vi "query.vi"(0 "object in":refnum<class "access_work.lvclass">, 1 "database":string(combo), 2 "table输入":string(combo), 3 "columns":string[](array[string]), 4 "condition":string, 5 "error in (no error)":errorcluster) -> (14 "object out":refnum<class "access_work.lvclass">, 15 "data":string[][](table), 16 "columns输出":string[](array[string]), 17 "拆分数据":bool, 19 "error out":errorcluster)   [LabVIEW 2016, in "access_work.lvclass"]
uses:
  access_work.lvclass
  <vilib>/Utility/sysdir.llb/System Directory Type.ctl
  <vilib>/addons/database/Connection.llb/DB Tools Open Connec (String).vi
  <vilib>/addons/database/_DB Variant To Data/Database Variant To Data.xnode
  <vilib>/addons/database/NI_Database_API.lvlib
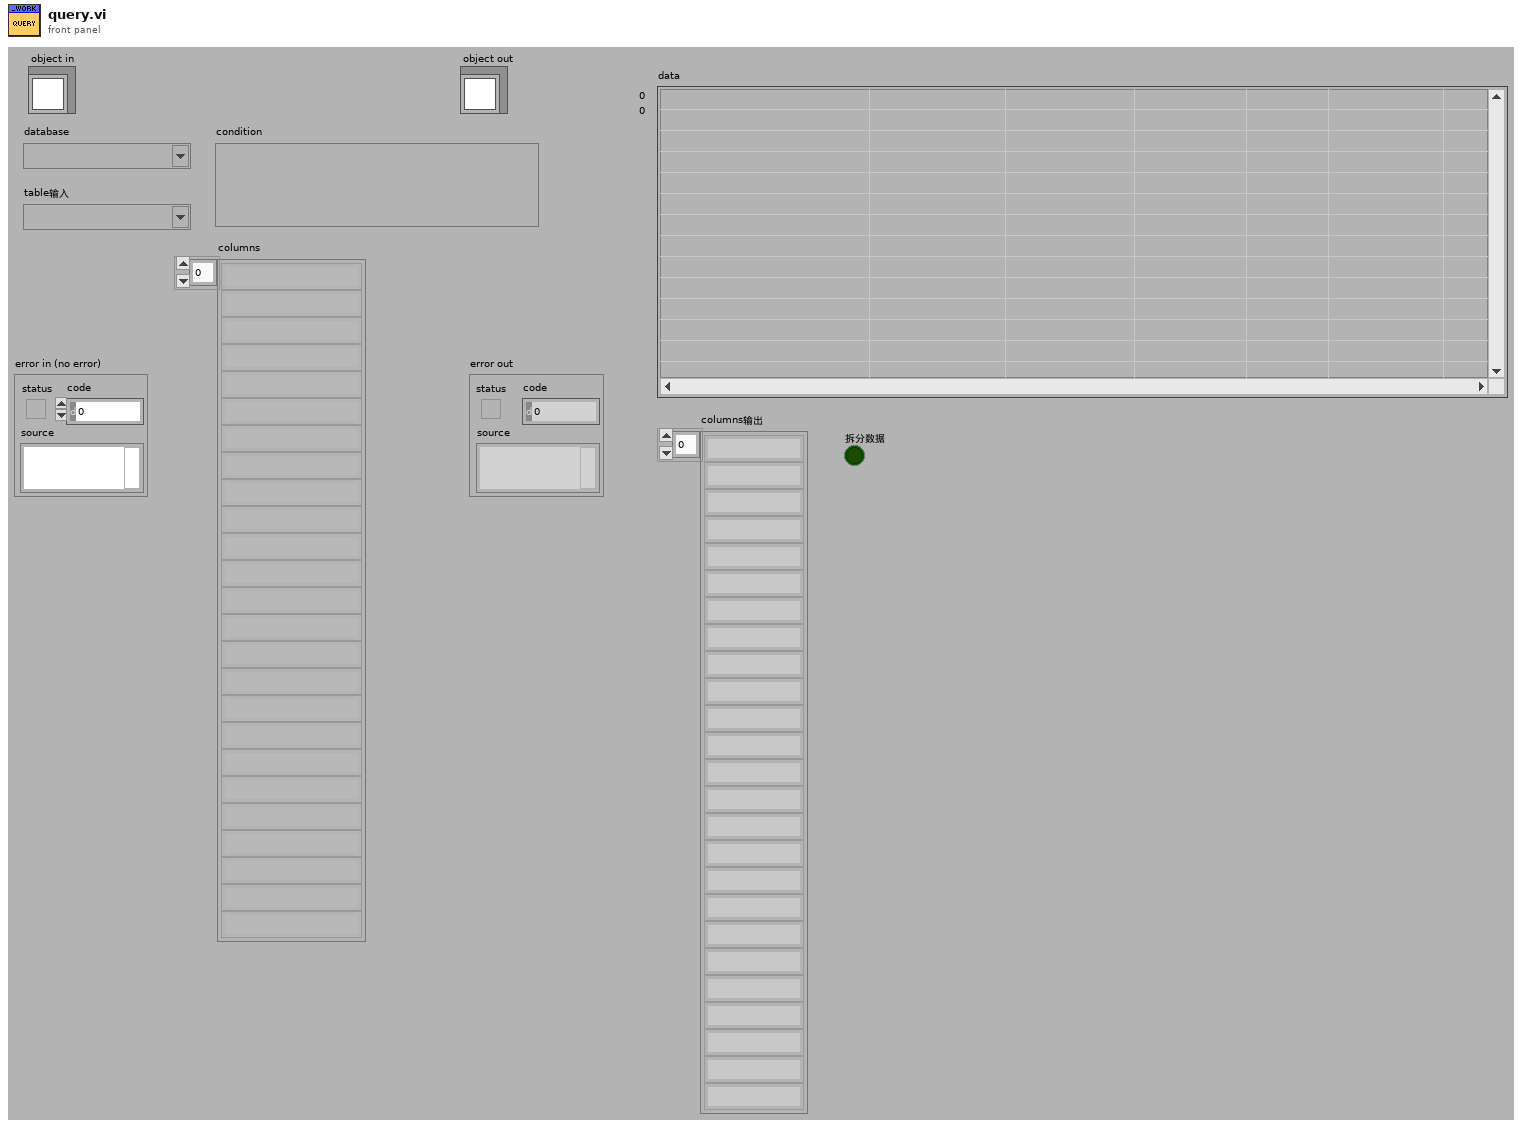
[diagram p1: front panel]
types:
  T1 = typedef "System Directory Type.ctl" = i32
  T2 = typedef "NI_Database_API.lvlib/Conn ObjectReference.ctl" = refnum<k1>
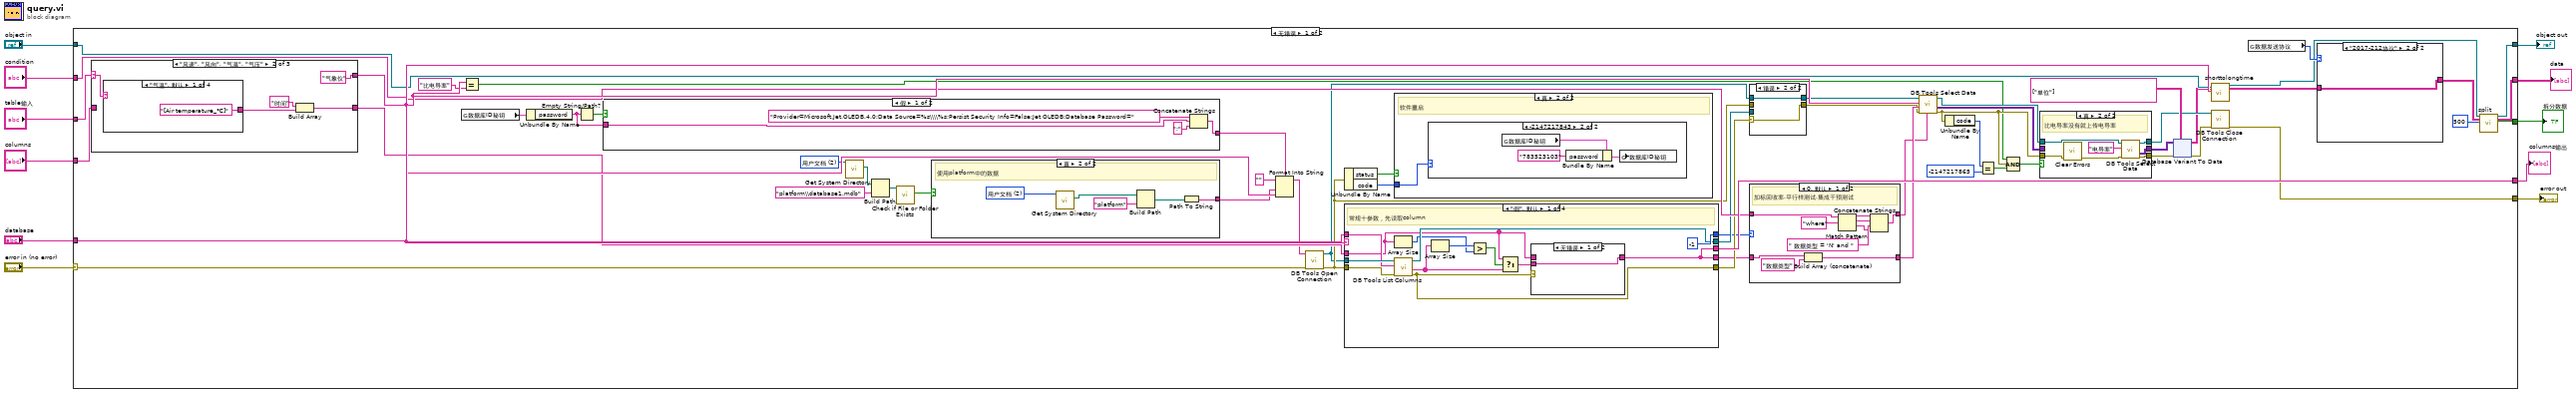
[diagram p0: block diagram]
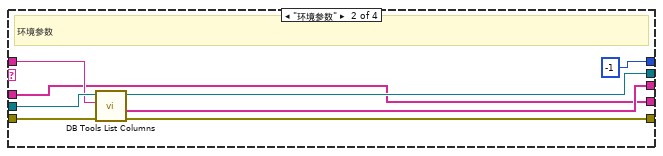
[diagram p6: hidden frame]
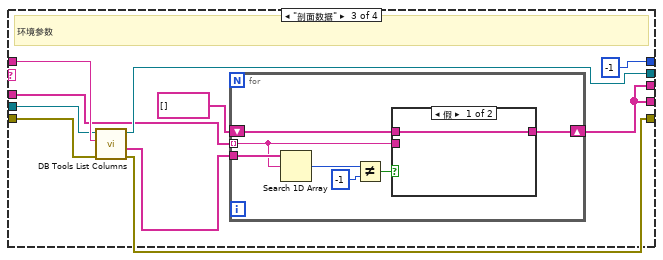
[diagram p7: hidden frame]
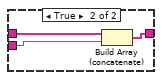
[diagram p8: hidden frame]
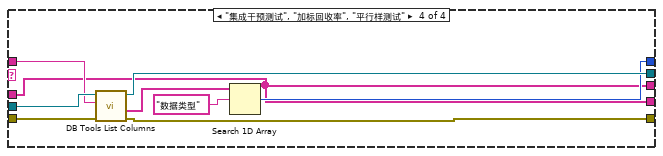
[diagram p9: hidden frame]
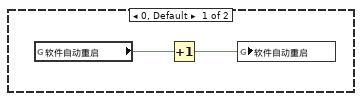
[diagram p11: hidden frame]
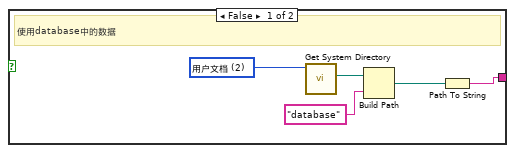
[diagram p12: hidden frame]
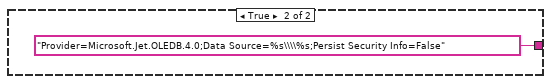
[diagram p13: hidden frame]
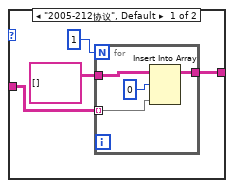
[diagram p14: hidden frame]
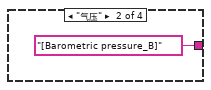
[diagram p16: hidden frame]
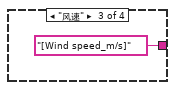
[diagram p17: hidden frame]
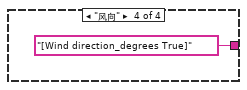
[diagram p18: hidden frame]
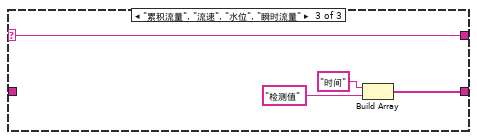
[diagram p19: hidden frame]
diagram:
  n1 = case shown="无错误" "error in (no error)" {
    selector: "error in (no error)" -> [w64 w238]
    tunnel: [w60 w238] -> w10
    tunnel: [w53 w237] -> w8
    tunnel: "object in" -> [w59 w237]
    tunnel: "table输入" -> [w68 _]
    tunnel: "columns" -> [w67 _]
    tunnel: "database" -> [w65 _]
    tunnel: [w63 _] -> w4
    tunnel: "condition" -> [w61 _]
    tunnel: [w52 _] -> w2
    tunnel: [w51 _] -> w1
    frame No Error {
      w45 = T1 2 items=["用户目录"=0, "用户桌面"=1, "用户文档"=2, "用户应用程序数据"=3, "用户设置"=4, "用户临时目录"=5, "公共文档"=6, "公共应用程序数据"=7, "公共设置"=8, "公共缓存"=13, "系统核心库"=9, "系统安装库"=10, "应用程序文件"=11, "启动盘根目录"=12] ("system directory type")
      n2 = case shown="\"风速\", \"风向\", \"气温\", \"气压\"" w68 {
        selector: w68 -> [w223 w227 w233]
        tunnel: [w223 "气象仪" w233] -> w66
        tunnel: w67 -> [w222 _ _]
        tunnel: [w222 w224 w235] -> w62
        frame "", Default {
        }
        frame "风速", "风向", "气温", "气压" {
          n3 = case shown="\"气温\", 默认" w227 {
            tunnel: ["[Air temperature_℃]" "[Barometric pressure_B]" "[Wind speed_m/s]" "[Wind direction_degrees True]"] -> w225
            frame "气温", Default {
            }
            frame "气压" {
            }
            frame "风速" {
            }
            frame "风向" {
            }
          }
          n4 = Build Array("时间", w225) -> (w224:string[])
        }
        frame "累积流量", "流速", "水位", "瞬时流量" {
          n5 = Build Array("时间", "检测值") -> (w235:string[])
        }
      }
      n6 = global read "外部交互全局.vi" "数据库ID秘钥"() -> (w49:cluster{"userID":string, "password":string})
      n7 = Equal?(x=w66, y="比电导率") -> (x = y?=w12:bool)
      n8 = Unbundle By Name(w49) -> ("password"=w47:string)
      n9 = Empty String/Path?(string/path=w47) -> (empty?=w48:bool)
      n10 = case shown="假" w48 {
        tunnel: [w208 "Provider=Microsoft.Jet.OLEDB.4.0;Data Source=%s\\\\%s;Persist Security Info=False" ("格式字符串")] -> w38
        tunnel: w47 -> [w211 _]
        frame False {
          n11 = Concatenate Strings("Provider=Microsoft.Jet.OLEDB.4.0;Data Source=%s\\\\%s;Persist Security Info=False;Jet OLEDB:Database Password=" ("格式字符串"), w211, ";" ("字符串")) -> (w208:string)
        }
        frame True {
        }
      }
      n12 = call <vilib>:"Get System Directory.vi"("system directory type"=w45) -> ("system directory"=w46:path)  [unwired: 10 in]
      n13 = Build Path(base path=w46, name or relative path="platform\\database1.mdb" ("condition")) -> (appended path=w44:path)
      n14 = call <vilib>:"Check if File or Folder Exists.vi"("path"=w44) -> ("file or folder exists?"=w42:bool)  [unwired: 8 in, 2 out]
      n15 = case shown="真" w42 {
        tunnel: [w198 w203] -> w39
        frame False {
          w201 = T1 2 items=["用户目录"=0, "用户桌面"=1, "用户文档"=2, "用户应用程序数据"=3, "用户设置"=4, "用户临时目录"=5, "公共文档"=6, "公共应用程序数据"=7, "公共设置"=8, "公共缓存"=13, "系统核心库"=9, "系统安装库"=10, "应用程序文件"=11, "启动盘根目录"=12] ("system directory type")
          # "使用database中的数据"
          n16 = call <vilib>:"Get System Directory.vi"("system directory type"=w201) -> ("system directory"=w200:path)  [unwired: 10 in]
          n17 = Build Path(base path=w200, name or relative path="database" ("condition")) -> (appended path=w202:path)
          n18 = Path To String(path=w202) -> (string=w198:string)
        }
        frame True {
          w207 = T1 2 items=["用户目录"=0, "用户桌面"=1, "用户文档"=2, "用户应用程序数据"=3, "用户设置"=4, "用户临时目录"=5, "公共文档"=6, "公共应用程序数据"=7, "公共设置"=8, "公共缓存"=13, "系统核心库"=9, "系统安装库"=10, "应用程序文件"=11, "启动盘根目录"=12] ("system directory type")
          # "使用platform中的数据"
          n19 = call <vilib>:"Get System Directory.vi"("system directory type"=w207) -> ("system directory"=w206:path)  [unwired: 10 in]
          n20 = Build Path(base path=w206, name or relative path="platform" ("condition")) -> (appended path=w204:path)
          n21 = Path To String(path=w204) -> (string=w203:string)
        }
      }
      n22 = Format Into String(format string=w38, initial string="" ("初始字符串"), w39, w65) -> (resulting string=w40:string)  [unwired: 1 in, 1 out]
      n23 = call-poly <vilib>:"DB Tools Open Connection.vi"("error in (no error)"=w64, "connection information"=w40) -> ("error out"=w34:errorcluster, "connection reference"=w32:T2)  [unwired: 6 in]
      n24 = Unbundle By Name(w34) -> ("status"=w37:bool, "code"=w36:i32)
      n25 = case shown="\"假\", 默认" w66 {
        tunnel: w32 -> [w150 w161 w169 w191]
        tunnel: w34 -> [w147 w160 w168 w189]
        tunnel: [w148 w159 w166 w188] -> w33
        tunnel: [w142 w158 w167 w187] -> w35
        tunnel: w66 -> [w149 w157 w170 w190]
        tunnel: [-1 ("index of element") -1 ("index of element") -1 ("index of element") w184] -> w31
        tunnel: w62 -> [w140 w154 w165 w183]
        tunnel: [w139 w155 w162 w183] -> w63
        tunnel: [w139 w154 w162 w183] -> w30
        frame "假", Default {
          # "常规十参数，先读取column"
          n26 = Array Size(array=w140) -> (size(s)=w144:i32)
          n27 = call <vilib>:"DB Tools List Columns.vi"("error in (no error)"=w147, "table"=w149, "connection reference"=w150) -> ("error out"=w142:errorcluster, "columns"=w143:string[], "connection reference out"=w148:T2)  [unwired: 1 in, 1 out]
          n28 = Array Size(array=w143) -> (size(s)=w145:i32)
          n29 = Greater?(x=w145, y=w144) -> (0:w146:bool)
          n30 = Select(t=w140, s=w146, f=w143) -> (s? t:f=w141:string[])
          n31 = case shown="无错误" w142 {
            tunnel: w141 -> [w152 _]
            tunnel: [w152 w153] -> w139
            tunnel: w140 -> [_ w153]
            frame No Error {
            }
            frame Error {
            }
          }
        }
        frame "环境参数" {
          # "环境参数"
          n32 = call <vilib>:"DB Tools List Columns.vi"("error in (no error)"=w160, "table"=w157, "connection reference"=w161) -> ("error out"=w158:errorcluster, "columns"=w155:string[], "connection reference out"=w159:T2)  [unwired: 1 in, 1 out]
        }
        frame "剖面数据" {
          # "环境参数"
          n33 = call <vilib>:"DB Tools List Columns.vi"("error in (no error)"=w168, "table"=w170, "connection reference"=w169) -> ("error out"=w167:errorcluster, "columns"=w164:string[], "connection reference out"=w166:T2)  [unwired: 1 in, 1 out]
          n34 = for {
            tunnel: w165 -> [w174] mode=indexing
            tunnel: w164 -> [w178]
            shift-right: [w172] -> w162
            shift-left: string[] [] -> [w175]
            n35 = Search 1D Array(1D array=w178, element=w174) -> (index of element=w177:i32)  [unwired: 1 in]
            n36 = Not Equal?(x=w177, y=-1) -> (x != y?=w173:bool)
            n37 = case shown="假" w173 {
              tunnel: w175 -> [w179 w182]
              tunnel: w174 -> [_ w181]
              tunnel: [w179 w180] -> w172
              frame False {
              }
              frame True {
                n38 = Build Array (concatenate)(w182, w181) -> (w180:string[])
              }
            }
          }
        }
        frame "集成干预测试", "加标回收率", "平行样测试" {
          n39 = call <vilib>:"DB Tools List Columns.vi"("error in (no error)"=w189, "table"=w190, "connection reference"=w191) -> ("error out"=w187:errorcluster, "columns"=w186:string[], "connection reference out"=w188:T2)  [unwired: 1 in, 1 out]
          n40 = Search 1D Array(1D array=w186, element="数据类型" ("元素")) -> (index of element=w184:i32)  [unwired: 1 in]
        }
      }
      n41 = case shown="真" w37 {
        tunnel: w36 -> [_ w192]
        frame False {
        }
        frame True {
          # "软件重启"
          n42 = case shown="-2147217843" w192 {
            frame 0, Default {
              n43 = global read "全局1.vi" "软件自动重启"() -> (w194:dbl)
              n44 = Increment(x=w194) -> (x+1=w193:dbl)
              n45 = global write "全局1.vi" "软件自动重启"(w193) -> ()
            }
            frame -2147217843 {
              n46 = global read "外部交互全局.vi" "数据库ID秘钥"() -> (w196:cluster{"userID":string, "password":string})
              n47 = Bundle By Name(cluster=w196, "password"="783523103") -> (w195:cluster{"userID":string, "password":string})
              n48 = global write "外部交互全局.vi" "数据库ID秘钥"(w195) -> ()
            }
          }
        }
      }
      n49 = case shown="错误" w35 {
        selector: w35 -> [_ w138]
        tunnel: w33 -> [w136 _]
        tunnel: [w136 w137] -> w16
        tunnel: w32 -> [_ w137]
        tunnel: [w135 w138] -> w15
        tunnel: w34 -> [w135 _]
        frame No Error {
        }
        frame Error {
        }
      }
      n50 = case "条件结构" shown="0, 默认" w31 {
        tunnel: w61 -> [w130 w133]
        tunnel: w30 -> [w132 w134]
        tunnel: [w124 w134] -> w17
        tunnel: [w123 w133] -> w14
        frame 0, Default {
          # "加标回收率,平行样测试,集成干预测试"
          n51 = Build Array (concatenate)(w132, "数据类型" ("元素")) -> (w124:string[])
          n52 = Match Pattern(string=w130, regular expression="where" ("正则表达式")) -> (before substring=w128:string, match substring=w127:string, after substring=w125:string)  [unwired: 1 in, 1 out]
          n53 = Concatenate Strings(w128, w127, " 数据类型 = 'N' and " ("字符串"), w125) -> (w123:string)
        }
        frame -1 {
        }
      }
      n54 = call <vilib>:"DB Tools Select Data.vi"("condition"=w14, "error in (no error)"=w15, "columns"=w17, "table"=w66, "connection reference"=w16) -> ("error out"=w21:errorcluster, "data"=w23:variant[][], "connection reference out"=w26:T2)  [unwired: 1 in]
      n55 = Unbundle By Name(w21) -> ("code"=w20:i32)
      n56 = Equal?(x=w20, y=-2147217865 ("code")) -> (x = y?=w18:bool)
      n57 = Compound Arithmetic op=AND ("复合运算")(w12, w21, w18) -> (w27:bool)
      n58 = case shown="真" w27 {
        tunnel: w26 -> [w71 w78]
        tunnel: [w71 w73] -> w25
        tunnel: [w70 w74] -> w24
        tunnel: w23 -> [w70 _]
        tunnel: w21 -> [w69 w76]
        tunnel: [w69 w72] -> w22
        frame False {
        }
        frame True {
          # "比电导率没有就上传电导率"
          n59 = call <vilib>:"Clear Errors.vi"("error in (no error)"=w76) -> ("error out"=w75:errorcluster)  [unwired: 5 in, 1 out]
          n60 = call <vilib>:"DB Tools Select Data.vi"("error in (no error)"=w75, "table"="电导率", "connection reference"=w78) -> ("error out"=w72:errorcluster, "data"=w74:variant[][], "connection reference out"=w73:T2)  [unwired: 3 in]
        }
      }
      n61 = xnode "Database Variant To Data"("database variant"=w24, "error in (no error)"=w22, "type"=string[][] [["单位"]]) -> ("data"=w13:string[][], "error out"=w28:errorcluster)
      n62 = call-dynamic "shorttolongtime.vi"("object in"=w59, "data"=w13, "table输入"=w66) -> ("object out"=w54:refnum<class "access_work.lvclass">, "输出数组"=w57:string[][])  [unwired: 14 in, 1 out]
      n63 = call <vilib>:"DB Tools Close Connection.vi"("error in (no error)"=w28, "connection reference"=w25) -> ("error out"=w60:errorcluster)  [unwired: 5 in]
      n64 = global read "断电保存全局.vi" "数据发送协议"() -> (w58:enum16{"2005-212协议", "2017-212协议"})
      n65 = case shown="\"2017-212协议\"" w58 {
        tunnel: w57 -> [w214 w221]
        tunnel: [w213 w221] -> w56
        frame "2005-212协议", Default {
          n66 = for {
            N: 1 -> [_]
            tunnel: string[][] [] ("data") -> [w220]
            tunnel: w214 -> [w219] mode=indexing
            tunnel: [w217] -> w213
            n67 = Insert Into Array(array=w220, index (row)=0 ("索引 (行)"), new element=w219) -> (w217:string[][])  [unwired: 1 in]
          }
        }
        frame "2017-212协议" {
        }
      }
      n68 = call-dynamic "split.vi"("object in"=w54, "输入数据"=w56, "拆分大小"=500) -> ("object out"=w53:refnum<class "access_work.lvclass">, "输出数组"=w52:string[][], "拆分数据"=w51:bool)  [unwired: 13 in, 1 out]
    }
    frame Error {
    }
  }
  "error out" <- w10
  "object out" <- w8
  "data" <- w2
  "columns输出" <- w4
  "拆分数据" <- w1
